vi "4-letteres_random_string_gen.vi"() -> (2 "4-letters random string":string)   [LabVIEW 2015]
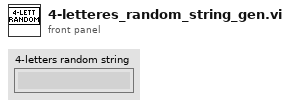
[diagram p1: front panel]
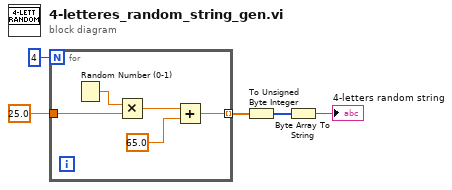
[diagram p0: block diagram]
diagram:
  n1 = for {
    N: 4 -> [_]
    tunnel: 25.0 ("y") -> [w9]
    tunnel: [w6] -> w3 mode=indexing
    n2 = Random Number (0-1)() -> (number: 0 to 1=w10:dbl)
    n3 = Multiply(x=w10, y=w9) -> (x*y=w8:dbl)
    n4 = Add(x=w8, y=65.0) -> (x+y=w6:dbl)
  }
  n5 = To Unsigned Byte Integer(number=w3) -> (unsigned 8bit integer=w2:u8[])
  n6 = Byte Array To String(unsigned byte array=w2) -> (string=→"4-letters random string":string)
